vi "esdaq_digitalDirectionMultiple.vi"(2 "esdaqErrorInp":errorcluster, 3 "ValueArray":bool[](array[boolean]), 4 "ChannelArray":u8[](array[numeric]), 5 "esdaqPortInp":refnum<visa-resource-name>) -> (0 "esdaqErrorOut":errorcluster, 1 "esdaqPortOut":refnum<visa-resource-name>)   [LabVIEW 2019]
panel:
  in  "tempString":string
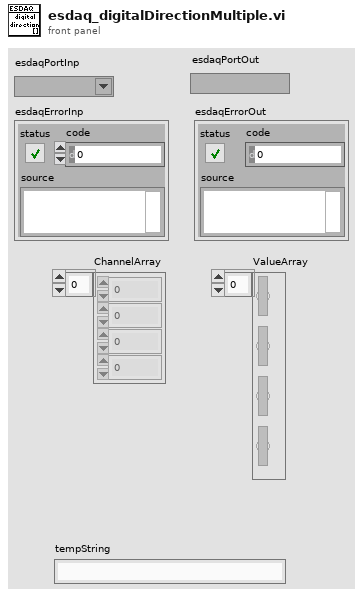
[diagram p1: front panel]
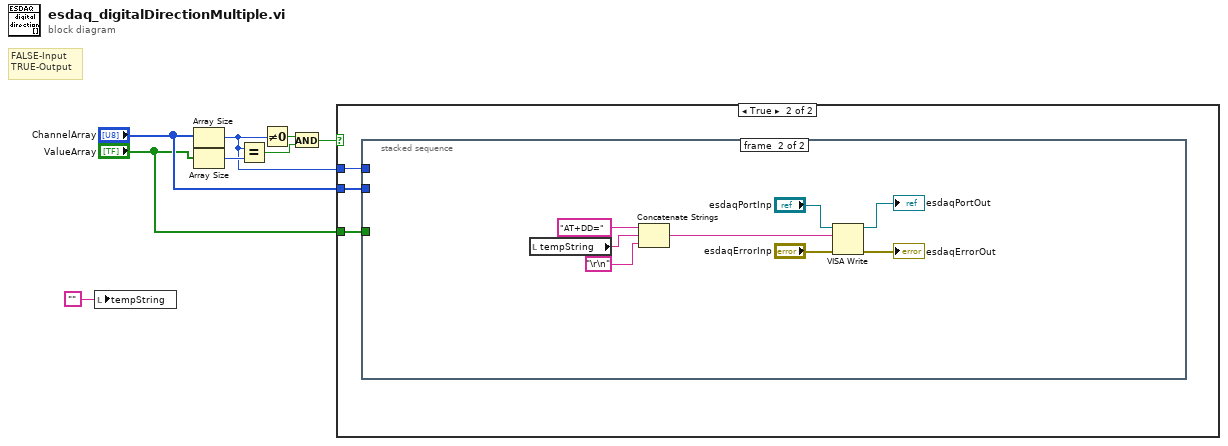
[diagram p0: block diagram]
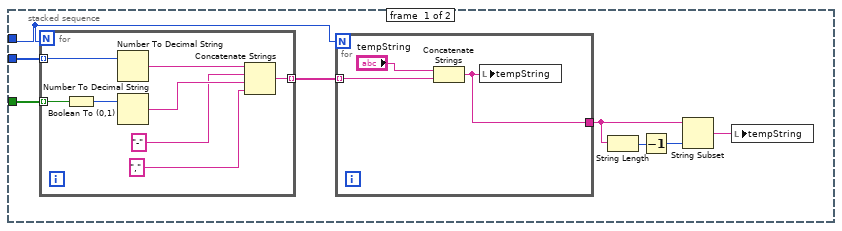
[diagram p3: hidden frame]
diagram:
  # "FALSE-Input\nTRUE-Output"
  n1 = local write "tempString"("") -> ()
  n2 = Array Size(array="ChannelArray") -> (size(s)=w4:i32)
  n3 = Array Size(array="ValueArray") -> (size(s)=w8:i32)
  n4 = Equal?(x=w4, y=w8) -> (x = y?=w6:bool)
  n5 = Not Equal To 0?(x=w4) -> (x != 0?=w7:bool)
  n6 = And(x=w7, y=w6) -> (x .and. y?=w5:bool)
  n7 = case shown="True" w5 {
    tunnel: w4 -> [_ w9]
    tunnel: "ChannelArray" -> [_ w11]
    tunnel: "ValueArray" -> [_ w10]
    frame False {
    }
    frame True {
      n8 = stacked-sequence {
        tunnel: w11 -> [w19 _]
        tunnel: w10 -> [w18 _]
        tunnel: w9 -> [w17 _]
        frame #0 {
          n9 = for {
            N: w17 -> [_]
            tunnel: w19 -> [w30] mode=indexing
            tunnel: w18 -> [w28] mode=indexing
            tunnel: [w23] -> w16 mode=indexing
            n10 = Boolean To (0,1)(Boolean=w28) -> (0, 1=w29:i16)
            n11 = Number To Decimal String(number=w30) -> (decimal integer string=w27:string)  [unwired: 1 in]
            n12 = Number To Decimal String(number=w29) -> (decimal integer string=w26:string)  [unwired: 1 in]
            n13 = Concatenate Strings(w27, "-", w26, ",") -> (w23:string)
          }
          n14 = for {
            N: w17 -> [_]
            tunnel: w16 -> [w22] mode=indexing
            tunnel: [w20] -> w12
            n15 = Concatenate Strings("tempString", w22) -> (w20:string)
            n16 = local write "tempString"(w20) -> ()
          }
          n17 = String Length(string=w12) -> (length=w15:i32)
          n18 = Decrement(x=w15) -> (x-1=w14:i32)
          n19 = String Subset(string=w12, length (rest)=w14) -> (substring=w13:string)  [unwired: 1 in]
          n20 = local write "tempString"(w13) -> ()
        }
        frame #1 {
          n21 = local read "tempString"() -> (w31:string)
          n22 = Concatenate Strings("AT+DD=", w31, "\r\n") -> (w34:string)
          n23 = VISA Write(VISA resource name="esdaqPortInp", write buffer=w34, error in (no error)="esdaqErrorInp") -> (VISA resource name out=→"esdaqPortOut":refnum<visa-resource-name>, error out=→"esdaqErrorOut":errorcluster)  [unwired: 1 out]
        }
      }
    }
  }
